vi "LWXPS_GroupPositionCorrectedProfilerGet.vi"(0 "XPS Reference IN":refnum<k24>, 1 "Group Name":string, 2 "Position X":dbl, 3 "Position Y":dbl, 5 "LabVIEW error IN":errorcluster) -> (14 "XPS Reference OUT":refnum<k24>, 15 "Returned error code":i32, 16 "Corrected Profiler Position X":dbl, 17 "Corrected Profiler Position Y":dbl, 18 "XPS Error String":string, 19 "LabVIEW error OUT":errorcluster)   [LabVIEW 2014]
uses:
  D:/XPSQ8_LabView_Library/Development/Source/Dll/Newport.XPS.CommandInterface.dll
  Dll/Newport.XPS.CommandInterface.dll
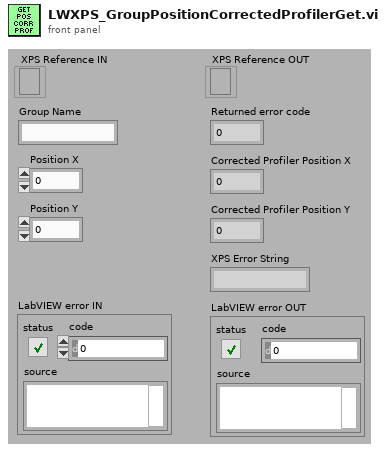
[diagram p1: front panel]
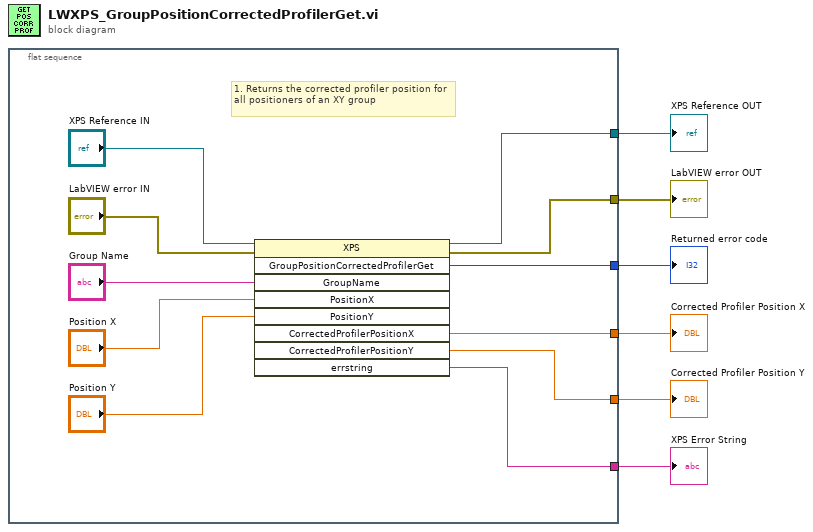
[diagram p0: block diagram]
diagram:
  n1 = flat-sequence {
    tunnel: [w12] -> w6
    tunnel: [w14] -> w5
    tunnel: [w16] -> w4
    tunnel: [w11] -> w1
    tunnel: [w10] -> w2
    tunnel: [w9] -> w3
    frame #0 {
      # "1. Returns the corrected profiler position for all positioners of an XY group"
      n2 = invoke class="XPS" method="GroupPositionCorrectedProfilerGet"(reference="XPS Reference IN", error in="LabVIEW error IN", "GroupName"="Group Name", "PositionX"="Position X", "PositionY"="Position Y") -> (reference out=w12:refnum<k24>, error out=w14:errorcluster, "GroupPositionCorrectedProfilerGet"=w16:i32, "CorrectedProfilerPositionX"=w10:dbl, "CorrectedProfilerPositionY"=w11:dbl, "errstring"=w9:string)  [unwired: 4 in, 3 out]
    }
  }
  "XPS Reference OUT" <- w6
  "LabVIEW error OUT" <- w5
  "Returned error code" <- w4
  "XPS Error String" <- w3
  "Corrected Profiler Position X" <- w2
  "Corrected Profiler Position Y" <- w1
